vi "WriteFPY.vi"(8 "error in (no error)":errorcluster, 10 "fail":i32, 11 "pass":i32) -> (0 "error out":errorcluster)   [LabVIEW 2013]
uses:
  <vilib>/Utility/file.llb/Write To Spreadsheet File (string).vi
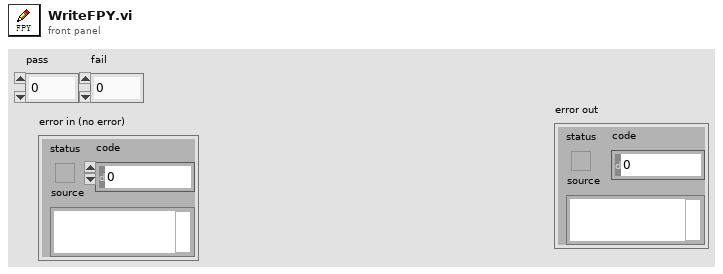
[diagram p1: front panel]
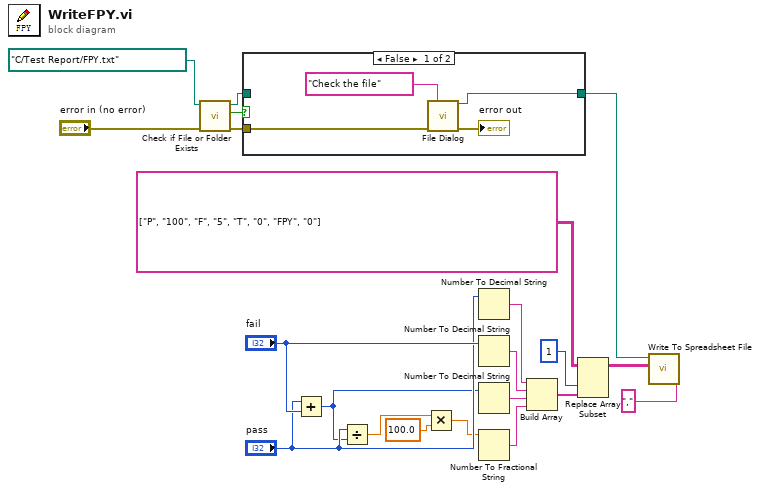
[diagram p0: block diagram]
diagram:
  n1 = call <vilib>:"Check if File or Folder Exists.vi"("error in (no error)"="error in (no error)", "path"=path "C:/Test Report/FPY.txt" ("start path")) -> ("error out"=w13:errorcluster, "file or folder exists?"=w18:bool, "dup path"=w17:path)  [unwired: 7 in]
  n2 = case shown="False" w18 {
    tunnel: w17 -> [_ w26]
    tunnel: [w25 w26] -> w16
    tunnel: w13 -> [w23 _]
    frame False {
      n3 = call "File Dialog"("prompt"="Check the file", "error in"=w23) -> ("selected path"=w25:path, "error out"=→"error out":errorcluster)  [unwired: 10 in, 2 out]
    }
    frame True {
    }
  }
  n4 = Add(x="pass", y="fail") -> (x+y=w1:i32)
  n5 = Divide(x="pass", y=w1) -> (x/y=w4:dbl)
  n6 = Multiply(x=w4, y=100.0) -> (x*y=w3:dbl)
  n7 = Number To Decimal String(number="pass") -> (decimal integer string=w10:string)  [unwired: 1 in]
  n8 = Number To Decimal String(number="fail") -> (decimal integer string=w9:string)  [unwired: 1 in]
  n9 = Number To Decimal String(number=w1) -> (decimal integer string=w7:string)  [unwired: 1 in]
  n10 = Number To Fractional String(number=w3) -> (F-format string=w8:string)  [unwired: 3 in]
  n11 = Build Array(w10, w9, w7, w8) -> (w11:string[])
  n12 = Replace Array Subset(array=string[][] [["P", "100"], ["F", "5"], ["T", "0"], ["FPY", "0"]] ("all rows"), new element=w11, index (col)=1 ("disabled index (col)")) -> (w12:string[][])  [unwired: 1 in]
  n13 = call-poly <vilib>:"Write To Spreadsheet File.vi"("delimiter (\\t)"="," ("delimiter (\\t)"), "2D data"=w12, "file path (dialog if empty)"=w16) -> ()  [unwired: 5 in, 1 out]
